vi "TecellaRCP.vi"(0 "TecellaClient in":refnum<class "TecellaClient.lvclass">, 5 "Name":string, 7 "method":string, 9 "Args":string[](array[string]), 11 "error in (no error)":errorcluster) -> (4 "TecellaClient out":refnum<class "TecellaClient.lvclass">, 6 "Data Returned":string, 15 "error out":errorcluster)   [LabVIEW 2009, in "TecellaClient.lvclass"]
uses:
  TecellaClient.lvclass
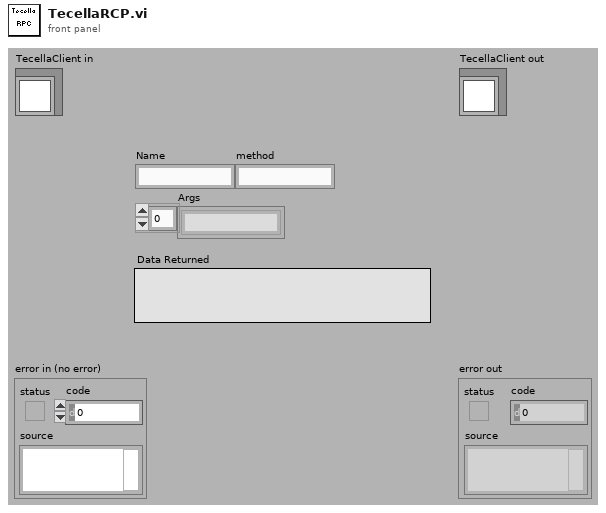
[diagram p1: front panel]
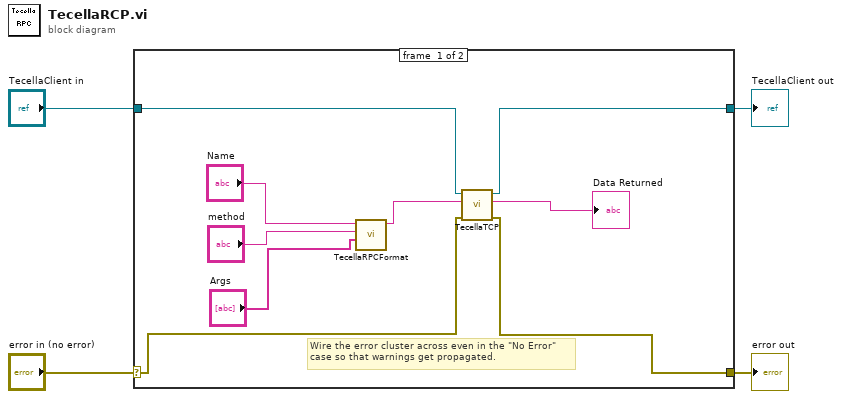
[diagram p0: block diagram]
diagram:
  n1 = case shown="No Error" "error in (no error)" {
    selector: "error in (no error)" -> [w6 w15]
    tunnel: [w5 w15] -> w3
    tunnel: [w13 w14] -> w1
    tunnel: "TecellaClient in" -> [w12 w14]
    frame #0 {
      # "Wire the error cluster across even in the \"No Error\"\ncase so that warnings get propagated."
      n2 = call "TecellaRPCFormat.vi"("Args"="Args", "method"="method", "Name"="Name") -> ("The RPC string"=w10:string)  [unwired: 8 in]
      n3 = call-dynamic "TecellaTCP.vi"("error in (no error)"=w6, "data in"=w10, "TecellaClient in"=w12) -> ("error out"=w5:errorcluster, "Data Returned"=→"Data Returned":string, "TecellaClient out"=w13:refnum<class "TecellaClient.lvclass">)  [unwired: 6 in]
    }
    frame #1 {
    }
  }
  "error out" <- w3
  "TecellaClient out" <- w1
